vi "Check If Aircraft Found.vi"(8 "Error In":errorcluster, 11 "Aircraft ID":u8) -> (0 "Error Out":errorcluster, 2 "Aircraft Index":i32, 3 "Aircraft Exists":bool)   [LabVIEW 2014]
uses:
  Aircraft Information/Sub VI/Get Aircraft Information.vi
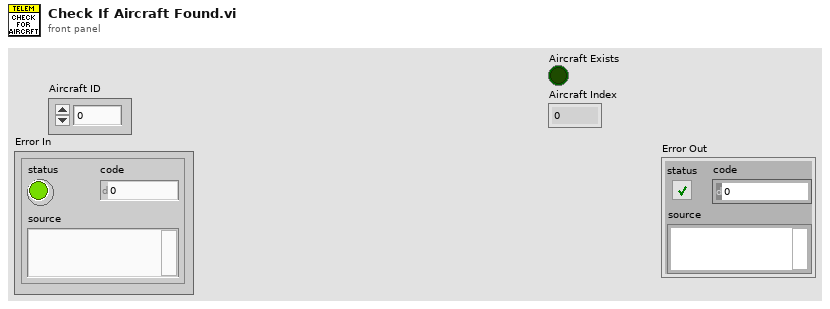
[diagram p1: front panel]
types:
  T1 = typedef "Drone Information.ctl" = cluster{"Heart Beat":bool, "Aircraft ID":u8, "Downlink Port":refnum<visa-resource-name>, "Tag ID":string, "System Status":string, "Base Mode":T2, "Armed/Disarmed":bool, "Battery Voltage":dbl, "Control Mode":T3, "Initialisation":u8, "Heart Beat Status":bool, "Uplink Port":refnum<visa-resource-name>, "UDP connection ID":refnum<k16>, "Connection Type":T4, "Mode":string, "UDP IP Address":string, "Mission Uploaded":bool}
  T2 = typedef "Base Mode.ctl" = cluster{"Custom Mode":bool, "Test Enabled":bool, "Autonomous Mode":bool, "Guided Mode":bool, "Stabilization Enabled":bool, "HIL Enabled":bool, "Manual Mode":bool, "Arm":bool}
  T3 = typedef "Aircraft Mode.ctl" = enum16{"Loiter", "Stabalise", "Failsafe", "Emergency Stop"}
  T4 = typedef "Telemetry Connection Type.ctl" = enum16{"Serial", "UDP", "TCP"}
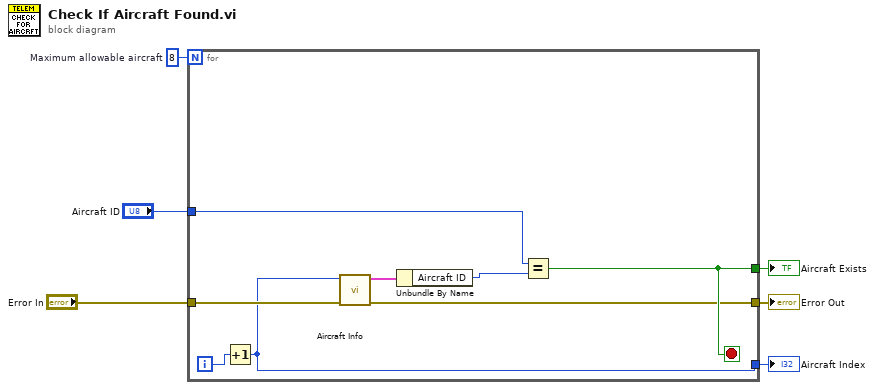
[diagram p0: block diagram]
diagram:
  w6 = 8  # Maximum allowable aircraft
  n1 = for {
    N: w6 -> [_]
    tunnel: "Error In" -> [w13]
    tunnel: "Aircraft ID" -> [w9]
    tunnel: [w10] -> w3
    tunnel: [w8] -> w2
    tunnel: [w7] -> w1
    i -> [w14]
    stop <- w10 stop-if-true
    n2 = Increment(x=w14) -> (x+1=w8:i32)
    n3 = call-poly "Aircraft Info.vi"("Error In"=w13, "Aircraft ID"=w8) -> ("Error Out"=w7:errorcluster, "Aircraft Information Out"=w12:T1)  [unwired: 8 in]
    n4 = Unbundle By Name(w12) -> ("Aircraft ID"=w11:u8)
    n5 = Equal?(x=w9, y=w11) -> (x = y?=w10:bool)
  }
  "Aircraft Exists" <- w3
  "Aircraft Index" <- w2
  "Error Out" <- w1
